vi "TestSampleMeasurement.vi"() -> ()   [LabVIEW 2019]
uses:
  enable_disable_enum_typedef.ctl
  MotorController.lvclass
panel:
  in  "SampleName":string
  in  "Exposure":u16
  in  "Serial Port":refnum<visa-resource-name>
  in  "Error In":errorcluster
  in  "Schedule File":path
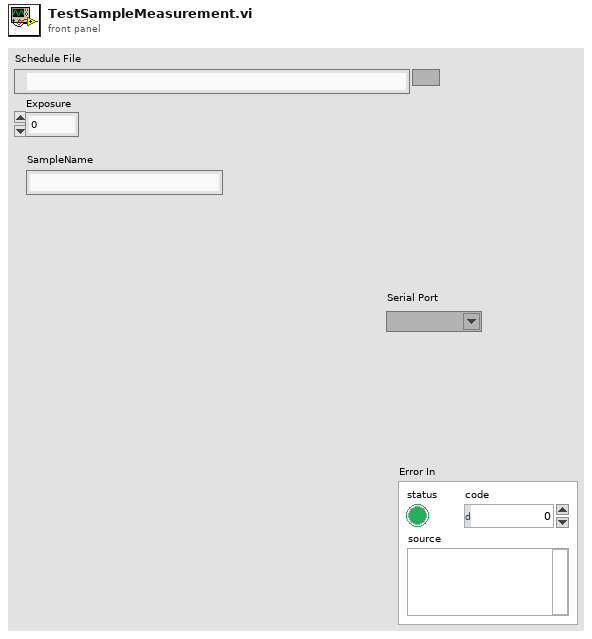
[diagram p1: front panel]
types:
  T1 = typedef "MotorController.lvclass/enable_disable_enum_typedef.ctl" = enum16{"Enable", "Disable"}
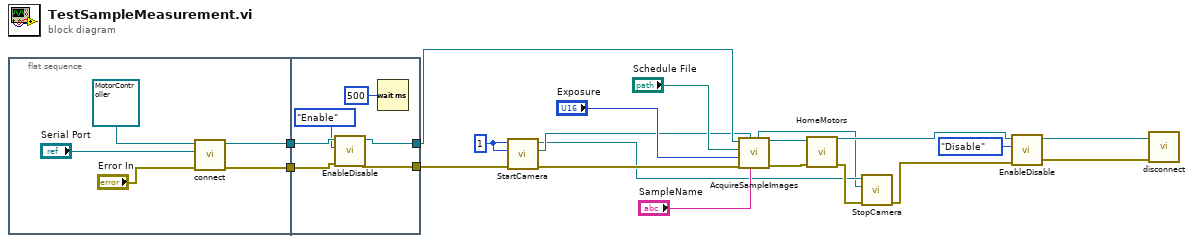
[diagram p0: block diagram]
diagram:
  w9 = u32 1 ("Gain")
  n1 = flat-sequence {
    tunnel: [w23] -> w19
    tunnel: [w22] -> w18
    tunnel: [w30] -> w8
    tunnel: w19 -> [w28]
    tunnel: w18 -> [w27]
    tunnel: [w29] -> w7
    frame #0 {
      n2 = call "connect.vi"("error in (no error)"="Error In", "Serial Port"="Serial Port", "MotorController in"=refnum<class "MotorController.lvclass"> refnum ("MotorController.lvclass")) -> ("error out"=w22:errorcluster, "MotorController out"=w23:refnum<class "MotorController.lvclass">)  [unwired: 7 in]
    }
    frame #1 {
      n3 = call "EnableDisable.vi"("error in (no error)"=w27, "Action"=enable_disable_enum_typedef."Enable", "MotorController in"=w28) -> ("error out"=w29:errorcluster, "MotorController out"=w30:refnum<class "MotorController.lvclass">)  [unwired: 7 in]
      n4 = Wait (ms)(milliseconds to wait=u32 500) -> ()  [unwired: 1 out]
    }
  }
  n5 = call "StartCamera.vi"("Error In"=w7, "ExposureTime_us"=w9, "Gain"=w9) -> ("Error Out"=w6:errorcluster, "TLCamera reference out"=w5:refnum<k24>, "TLCameraSDK reference out"=w2:refnum<k24>)  [unwired: 6 in]
  n6 = call "AcquireSampleImages.vi"("SampleName"="SampleName", "TLCamera reference in"=w5, "Error In"=w6, "Exposure"="Exposure", "Schedule File"="Schedule File", "MotorController in"=w8) -> ("Error Out"=w12:errorcluster, "MotorController out"=w13:refnum<class "MotorController.lvclass">, "TLCamera reference out"=w1:refnum<k24>)  [unwired: 3 in]
  n7 = call "HomeMotors.vi"("error in (no error)"=w12, "MotorController in"=w13) -> ("error out"=w4:errorcluster, "MotorController out"=w11:refnum<class "MotorController.lvclass">)  [unwired: 8 in]
  n8 = call "StopCamera.vi"("Error In"=w4, "TLCamera reference"=w1, "TLCameraSDK reference"=w2) -> ("Error Out"=w3:errorcluster)  [unwired: 8 in]
  n9 = call "EnableDisable.vi"("error in (no error)"=w3, "Action"=enable_disable_enum_typedef."Disable", "MotorController in"=w11) -> ("error out"=w15:errorcluster, "MotorController out"=w16:refnum<class "MotorController.lvclass">)  [unwired: 7 in]
  n10 = call "disconnect.vi"("error in (no error)"=w15, "MotorController in"=w16) -> ()  [unwired: 8 in, 2 out]
